vi "sweep_delay.vi"(11 "Command":string) -> (3 "Delay Time":dbl)   [LabVIEW 2015]
panel:
  out "Bias Step":dbl
  out "Bias Stop":dbl
  out "Bias Start":dbl
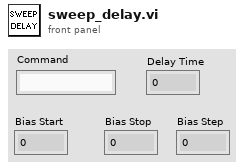
[diagram p1: front panel]
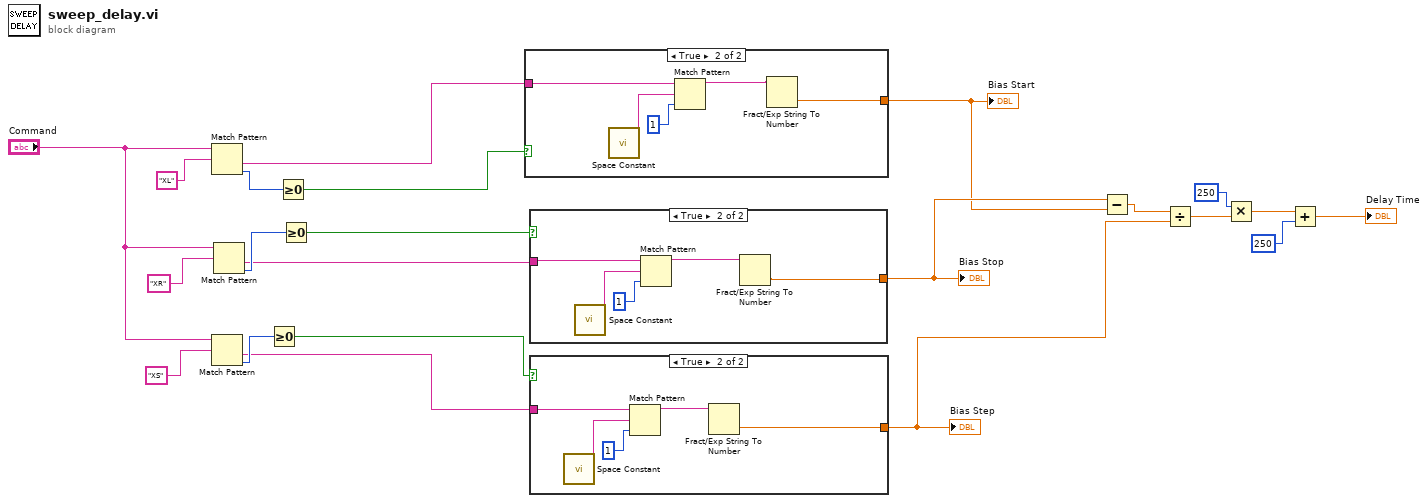
[diagram p0: block diagram]
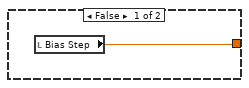
[diagram p2: hidden frame]
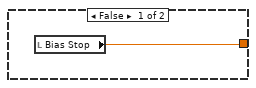
[diagram p3: hidden frame]
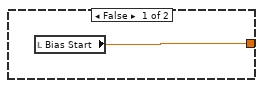
[diagram p4: hidden frame]
diagram:
  n1 = Match Pattern(string="Command", regular expression="XL") -> (after substring=w14:string, offset past match=w19:i32)  [unwired: 1 in, 2 out]
  n2 = Match Pattern(string="Command", regular expression="XS") -> (after substring=w10:string, offset past match=w16:i32)  [unwired: 1 in, 2 out]
  n3 = Match Pattern(string="Command", regular expression="XR") -> (after substring=w12:string, offset past match=w20:i32)  [unwired: 1 in, 2 out]
  n4 = Greater Or Equal To 0?(x=w16) -> (x >= 0?=w11:bool)
  n5 = Greater Or Equal To 0?(x=w19) -> (x >= 0?=w15:bool)
  n6 = Greater Or Equal To 0?(x=w20) -> (x >= 0?=w13:bool)
  n7 = case shown="True" w15 {
    tunnel: w14 -> [_ w26]
    tunnel: [w23 w24] -> w8
    frame False {
      n8 = local read "Bias Start"() -> (w23:dbl)
    }
    frame True {
      n9 = call <vilib>:"Space Constant.vi"() -> ("String"=w27:string)
      n10 = Match Pattern(string=w26, regular expression=w27, offset (0)=1) -> (before substring=w25:string)  [unwired: 3 out]
      n11 = Fract/Exp String To Number(string=w25) -> (number=w24:dbl)  [unwired: 3 in, 1 out]
    }
  }
  "Bias Start" <- w8
  n12 = case shown="True" w13 {
    tunnel: w12 -> [_ w32]
    tunnel: [w29 w30] -> w9
    frame False {
      n13 = local read "Bias Stop"() -> (w29:dbl)
    }
    frame True {
      n14 = call <vilib>:"Space Constant.vi"() -> ("String"=w34:string)
      n15 = Match Pattern(string=w32, regular expression=w34, offset (0)=1) -> (before substring=w31:string)  [unwired: 3 out]
      n16 = Fract/Exp String To Number(string=w31) -> (number=w30:dbl)  [unwired: 3 in, 1 out]
    }
  }
  "Bias Stop" <- w9
  n17 = case shown="True" w11 {
    tunnel: w10 -> [_ w38]
    tunnel: [w35 w36] -> w6
    frame False {
      n18 = local read "Bias Step"() -> (w35:dbl)
    }
    frame True {
      n19 = call <vilib>:"Space Constant.vi"() -> ("String"=w40:string)
      n20 = Match Pattern(string=w38, regular expression=w40, offset (0)=1) -> (before substring=w37:string)  [unwired: 3 out]
      n21 = Fract/Exp String To Number(string=w37) -> (number=w36:dbl)  [unwired: 3 in, 1 out]
    }
  }
  "Bias Step" <- w6
  n22 = Subtract(x=w9, y=w8) -> (x-y=w7:dbl)
  n23 = Divide(x=w7, y=w6) -> (x/y=w5:dbl)
  n24 = Multiply(x=250, y=w5) -> (x*y=w3:dbl)
  n25 = Add(x=w3, y=250) -> (x+y=→"Delay Time":dbl)
